vi "Normal PDF.vi"(9 "std":dbl=1.0, 10 "mean":dbl, 11 "x":dbl) -> (0 "error":i32, 3 "pdf(x)":dbl=0.3989422804014327)   [LabVIEW 2014, in "NI_Gmath.lvlib"]
doc: "Computes the continuous probability density function (PDF) of various distributions. You must manually select the polymorphic instance to use."
uses:
  NI_Gmath.lvlib
  st_error_code.ctl
panel:
  # "Normal PDF"
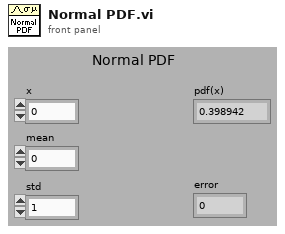
[diagram p1: front panel]
types:
  T1 = typedef "NI_Gmath.lvlib/st_error_code.ctl" = i32
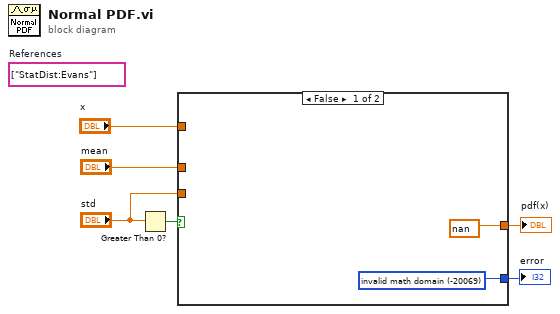
[diagram p0: block diagram]
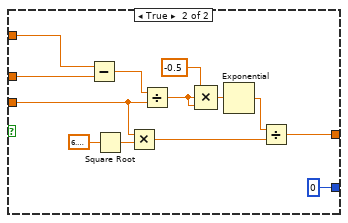
[diagram p2: hidden frame]
diagram:
  (unwired) string[] ["StatDist:Evans"]  # References
  n1 = Greater Than 0?(x="std") -> (x > 0?=w6:bool)
  n2 = case shown="False" w6 {
    tunnel: "std" -> [_ w13]
    tunnel: [w7 0 ("invalid math domain")] -> w4
    tunnel: [nan w9] -> w3
    tunnel: "x" -> [_ w19]
    tunnel: "mean" -> [_ w20]
    frame False {
      w7 = T1 -20069 items=["invalid math domain"=-20069, "Fourier interpolation size m >= n"=-20070, "empty array"=-20003] ("stat interp error code")
    }
    frame True {
      n3 = Subtract(x=w19, y=w20) -> (x-y=w18:dbl)
      n4 = Square Root(x=6.283185307179586) -> (sqrt(x)=w14:dbl)
      n5 = Multiply(x=w13, y=w14) -> (x*y=w11:dbl)
      n6 = Divide(x=w18, y=w13) -> (x/y=w16:dbl)
      n7 = Compound Arithmetic op=MULTIPLY(-0.5, w16, w16) -> (w12:dbl)
      n8 = Exponential(1:w12) -> (0:w10:dbl)
      n9 = Divide(x=w10, y=w11) -> (x/y=w9:dbl)
    }
  }
  "pdf(x)" <- w3
  "error" <- w4
